vi "State_Machine.vi"(8 "error in (no error)":errorcluster caption="entrée d'erreur (pas d'erreur)", 11 "Get_Voltage en entrée":refnum<class "Get_Key_DB_AIS.lvclass">) -> (0 "error out":errorcluster caption="sortie d'erreur", 2 "Json_String":string, 3 "Get_Voltage en sortie":refnum<class "Get_Key_DB_AIS.lvclass">)   [LabVIEW 2020, in "Library Test.lvlib" / "Get_Key_DB_AIS.lvclass"]
uses:
  Get_Key_DB_AIS.lvclass
  C:/Users/ngarcin/OneDrive - Altyor/Standard TB/Suite TB45/Class/Test/Find_SN_In_Database/Find_SN_In_Database.lvclass
  C:/Users/ngarcin/OneDrive - Altyor/Standard TB/Suite TB45/Class/Test/Test (Default)/Test (Default).lvclass
  Commun VI/TypeDef/Variable Printable.ctl
  JSON API/JSON Value/Set from JSON string.vi
  JSON API/JSON Value/JSON Value.lvclass
  Find_SN_In_Database/Find_SN_In_Database.lvclass
  Commun VI/Library Commun.lvlib
  JSON API/Variant JSON/Variant JSON.lvlib
  JSON API/Get Polymorphic/JSON GetSet.lvlib
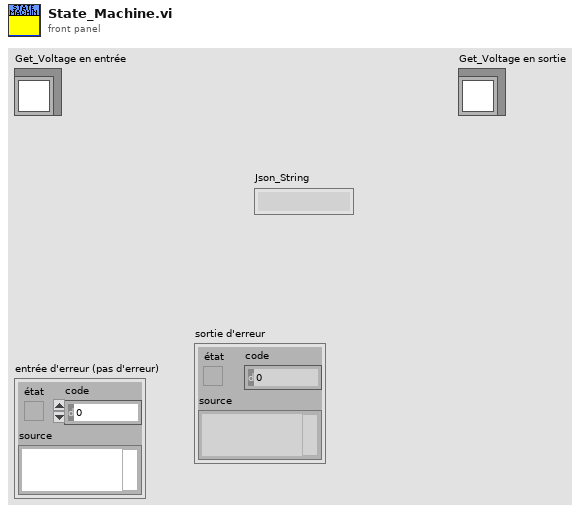
[diagram p1: front panel]
types:
  T1 = typedef "Variable Printable.ctl" = string
  T2 = enum16{"Get Variable", "Get All Variables", "Set Variable", "Delete Variable", "Delete All Variable"}
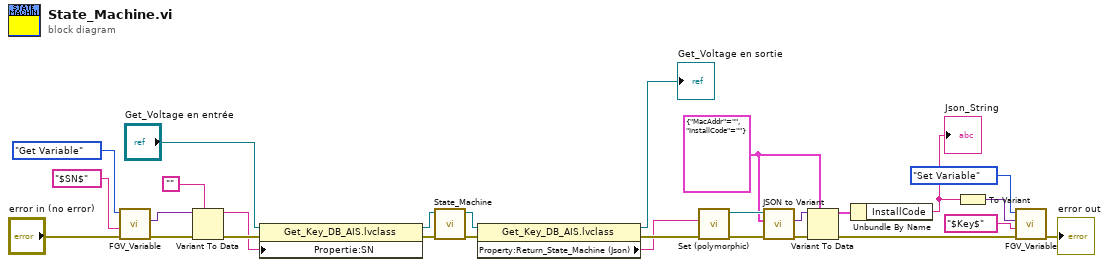
[diagram p0: block diagram]
diagram:
  w15 = cluster{"MacAddr":string, "InstallCode":string} {"MacAddr"="", "InstallCode"=""}
  n1 = call "FGV_Variable.vi"("error in (no error)"="error in (no error)", "Variable"=T1 "$SN$", "Function"=T2."Get Variable") -> ("error out"=w7:errorcluster, "Data Out"=w6:variant)  [unwired: 6 in, 1 out]
  n2 = Variant To Data(error in=w7, type="", Variant=w6) -> (data=w2:string, error out=w3:errorcluster)
  n3 = property class="Get_Key_DB_AIS.lvclass"(reference="Get_Voltage en entrée", error in=w3, "Propertie:SN"=w2) -> (reference out=w10:refnum<class "Get_Key_DB_AIS.lvclass">, error out=w9:errorcluster)
  n4 = call-parent "State_Machine.vi"("error in (no error)"=w9, "Generate_SN en entrée"=w10) -> ("error out"=w23:errorcluster, "Generate_SN en sortie"=w22:refnum<class "Get_Key_DB_AIS.lvclass">)  [unwired: 7 in, 1 out]
  n5 = property class="Get_Key_DB_AIS.lvclass"(reference=w22, error in=w23) -> (reference out=→"Get_Voltage en sortie":refnum<class "Get_Key_DB_AIS.lvclass">, error out=w17:errorcluster, "Property:Return_State_Machine (Json)"=w16:string)
  n6 = call-poly "Set (polymorphic).vi"("error in (no error)"=w17, "JSON stream"=w16) -> ("error out"=w20:errorcluster, "JSON Value out"=w18:refnum<class "JSON Value.lvclass">)  [unwired: 7 in, 1 out]
  n7 = call "JSON to Variant.vi"("error in (no error)"=w20, "Variant (Data Type)"=w15, "JSON Value"=w18) -> ("error out"=w19:errorcluster, "Variant out"=w21:variant)  [unwired: 7 in]
  n8 = Variant To Data(error in=w19, type=w15, Variant=w21) -> (data=w14:cluster{"MacAddr":string, "InstallCode":string}, error out=w12:errorcluster)
  n9 = Unbundle By Name(w14) -> ("InstallCode"=w13:string)
  "Json_String" <- w13
  n10 = To Variant(anything=w13) -> (Variant=w24:variant)
  n11 = call "FGV_Variable.vi"("error in (no error)"=w12, "Variable"=T1 "$Key$" ("Variable Printable"), "Data In"=w24, "Function"=T2."Set Variable") -> ("error out"=→"error out":errorcluster)  [unwired: 5 in, 2 out]
